vi "Exemple_Metrics_Hinge_Loss.vi"() -> ()   [LabVIEW 2020]
uses:
  Objet/3 - Model selection and evaluation/3.3 - Metrics and scoring/hinge_loss/Hinge_Loss.vi
panel:
  out "Score":string
  out "error out":errorcluster caption="sortie d'erreur"
  in  "error in (no error)":errorcluster caption="entrée d'erreur (pas d'erreur)"
  in  "hinge_loss":cluster{"labels":i32[], "sample_weight":dbl[]}
  in  "pred_decision":string[][](array[string])=[["-2.181772618720317"], ["2.3636168365944212"], ["0.09092210893705227"]]
  in  "y_true":string[][](array[string])=[["-1"], ["1"], ["1"]]
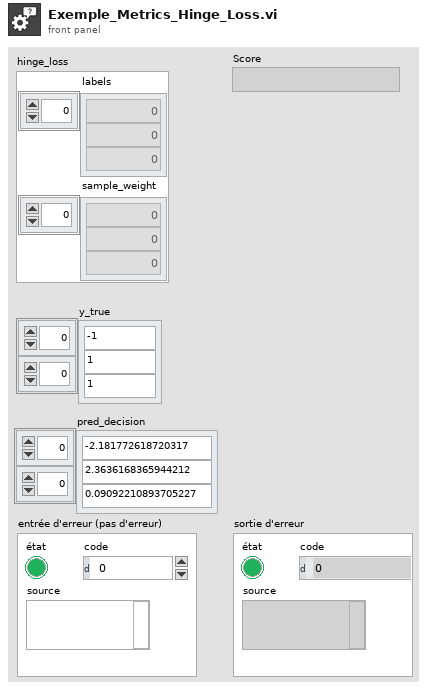
[diagram p1: front panel]
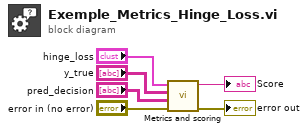
[diagram p0: block diagram]
diagram:
  n1 = call-poly "Metrics and scoring.vi"("error in (no error)"="error in (no error)", "pred_decision"="pred_decision", "y_true"="y_true", "hinge_loss"="hinge_loss") -> ("error out"=→"error out":errorcluster, "Score"=→"Score":string)  [unwired: 6 in]
